vi "freqout --monitor -- format.vi"(7 "freqout action":enum16{"header", "one line", "one"}(ring)=enum."one line", 8 "segments string":string="Segments:{}", 9 "timestamp":timestamp, 10 "temperature":dbl, 11 "lorentzian":T1={"Amplitude"=-1.0311345636926572, "omega(0)"=-1.0311345636926572, "Gamma"=-1.0311345636926572, "phase"=-1.0311345636926572, "Q"=-1.0311345636926572, "Norm  Ampl"=-1.0311345636926572, "z (inf)"=-1.0311345636926572+0.0i, "4corners"={"z (-pi/2)"=-1.0311345636926572+0.5736824521422934i, "z(inf)"=-0.5200164984937075+1.0975277942502903i, "z (pi/2)"=-1.0311345636926572+0.5736824521422934i, "z center"=-0.5136528600391839+0.580046090596817i, "z(0)"=-0.5200164984937075+1.0975277942502903i, "radius"=-1.0311345636926572}} {"z (inf)" format="%#9_9f"; "Q" format="%#9_9f"; "phase" format="%#9_9f"; "Gamma" format="%#9_9f"; "omega(0)" format="%#9_9f"}) -> (0 "output string":string)   [LabVIEW 2010]
uses:
  lorentzian.ctl
  circle corners.ctl
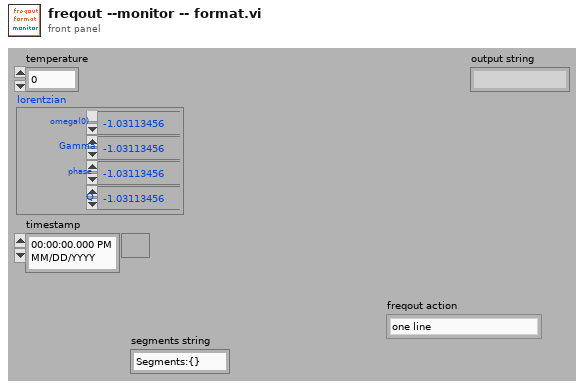
[diagram p1: front panel]
types:
  T1 = typedef "lorentzian.ctl" = cluster{"Amplitude":dbl, "omega(0)":dbl, "Gamma":dbl, "phase":dbl, "Q":dbl, "Norm  Ampl":dbl, "z (inf)":cdb, "4corners":T2}
  T2 = typedef "circle corners.ctl" = cluster{"z (-pi/2)":cdb, "z(inf)":cdb, "z (pi/2)":cdb, "z center":cdb, "z(0)":cdb, "radius":dbl}
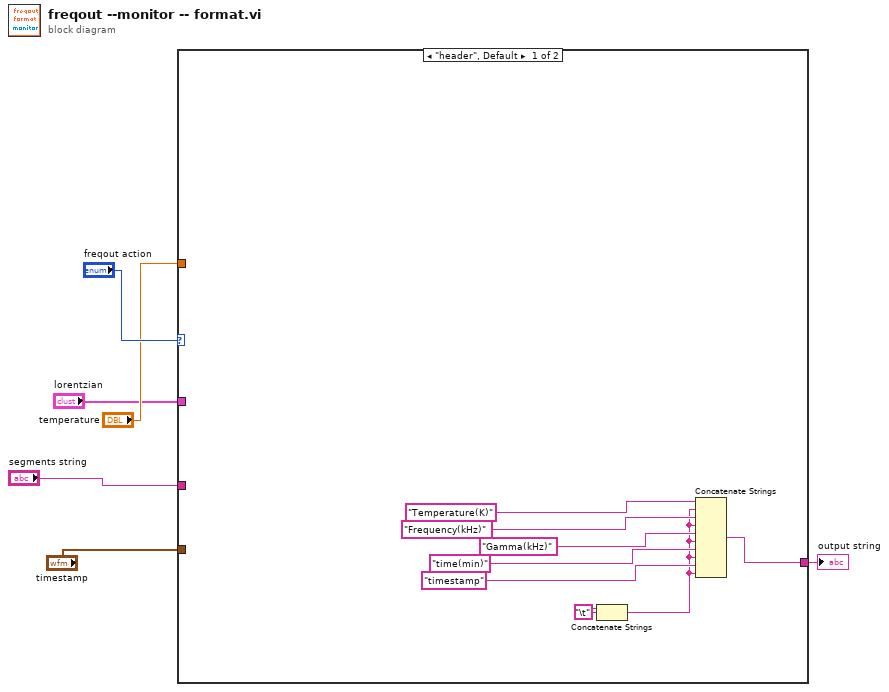
[diagram p0: block diagram]
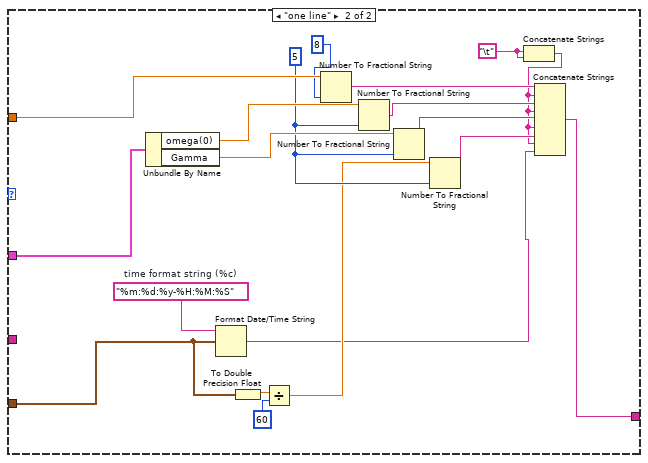
[diagram p2: hidden frame]
diagram:
  n1 = case shown="\"header\", Default" "freqout action" {
    tunnel: [w7 w20] -> w1
    tunnel: "segments string" -> [_ _]
    tunnel: "temperature" -> [_ w33]
    tunnel: "lorentzian" -> [_ w32]
    tunnel: "timestamp" -> [_ w17]
    frame "header", Default {
      w9 = "\t"
      n2 = Concatenate Strings(w9, w9) -> (w8:string)
      n3 = Concatenate Strings("Temperature(K)", w8, "Frequency(kHz)", w8, "Gamma(kHz)", w8, "time(min)", w8, "timestamp", w8) -> (w7:string)
    }
    frame "one line" {
      w22 = "%m:%d:%y-%H:%M:%S"  # time format string (%c)
      w27 = "\t"
      w24 = i16 5 ("precision (6)")
      n4 = Unbundle By Name(w32) -> ("omega(0)"=w30:dbl, "Gamma"=w28:dbl)
      n5 = Format Date/Time String(time format string (%c)=w22, seconds (now)=w17) -> (date/time string=w15:string)  [unwired: 1 in]
      n6 = To Double Precision Float(number=w17) -> (double precision float=w19:dbl)
      n7 = Divide(x=w19, y=60) -> (x/y=w16:dbl)
      n8 = Number To Fractional String(number=w33, precision (6)=i16 8) -> (F-format string=w31:string)  [unwired: 2 in]
      n9 = Number To Fractional String(number=w30, precision (6)=w24) -> (F-format string=w29:string)  [unwired: 2 in]
      n10 = Number To Fractional String(number=w28, precision (6)=w24) -> (F-format string=w25:string)  [unwired: 2 in]
      n11 = Number To Fractional String(number=w16, precision (6)=w24) -> (F-format string=w26:string)  [unwired: 2 in]
      n12 = Concatenate Strings(w27, w27) -> (w23:string)
      n13 = Concatenate Strings(w31, w23, w29, w23, w25, w23, w26, w23, w15) -> (w20:string)
    }
  }
  "output string" <- w1
